vi "IAmGLF-SendToStandaloneProcess.vi"(8 "error in (no error)":errorcluster, 10 "Class Return Notifier":refnum<notifier>, 11 "IUseDVRHandler in":refnum<class "IUseDVRHandler.lvclass">) -> (0 "error out":errorcluster, 3 "IUseDVRHandler out":refnum<class "IUseDVRHandler.lvclass">)   [LabVIEW 2024, in "GLF.lvlib" / "IUseDVRHandler.lvclass"]
doc: "<B>Summary</B>\nUsed to send <B>IAmGLF</B> along with <B>Data</B> to a standalone entity in order for it to create the class internal DVR.\n\n<B>Default Behavior</B>\nIf not overriden, this will <B>TODO</B>\n\n<B>Details</B>\nThis is done that way because LabVIEW automatically releases references created by VIs (or their callers) that are no longer running. So we must rely on an another asych process to be sure the DVR is not deleted."
uses:
  IUseDVRHandler.lvclass
  IAmGLF/IAmGLF.lvclass
  DVRHandler/DVRHandler.lvlib
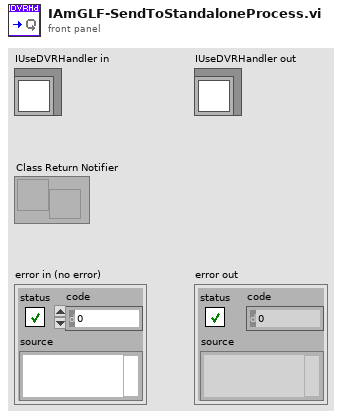
[diagram p1: front panel]
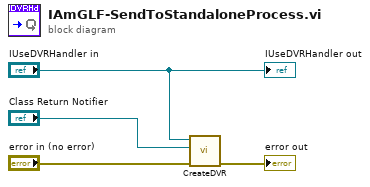
[diagram p0: block diagram]
diagram:
  n1 = call "CreateDVR.vi"("error in (no error)"="error in (no error)", "IAmGLF Return Notifier"="Class Return Notifier", "IAmGLF To Create DVR"="IUseDVRHandler in") -> ("error out"=→"error out":errorcluster)  [unwired: 8 in]
  "IUseDVRHandler out" <- "IUseDVRHandler in"
